vi "Add FPGA Channels.vi"(7 "error in (no error)":errorcluster, 9 "User defined IOVs":T1(array[cluster]), 10 "Item Ref in":T2 format="%.0x") -> (0 "error out":errorcluster, 3 "Item Ref out":T2 format="%.0x")   [LabVIEW 2019, in "SEECD System Explorer.lvlib"]
uses:
  SEECD System Explorer.lvlib
  <vilib>/NI VeriStand/Custom Device API/Custom Device Item Ref.ctl
  <vilib>/NI VeriStand/Custom Device API/Custom Device Channel Type.ctl
  <vilib>/NI VeriStand/Custom Device API/Custom Device API.lvlib
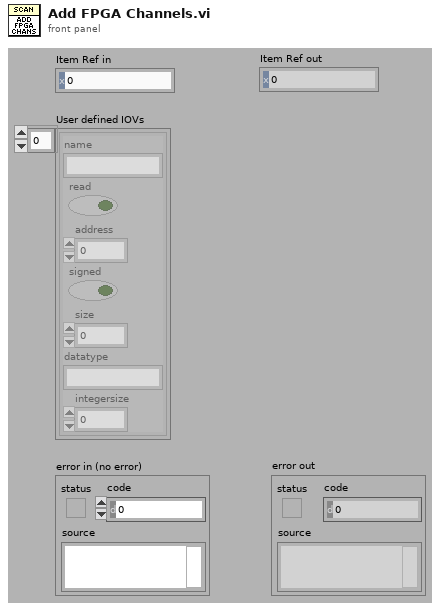
[diagram p1: front panel]
types:
  T1 = cluster{"name":string, "read":bool, "address":u32, "signed":bool, "size":u32, "datatype":string, "integersize":i32}[]
  T2 = typedef "Custom Device API.lvlib/Custom Device Item Ref.ctl" = u64
  T3 = typedef "Custom Device API.lvlib/Custom Device Channel Type.ctl" = enum16{"Input", "Output"}
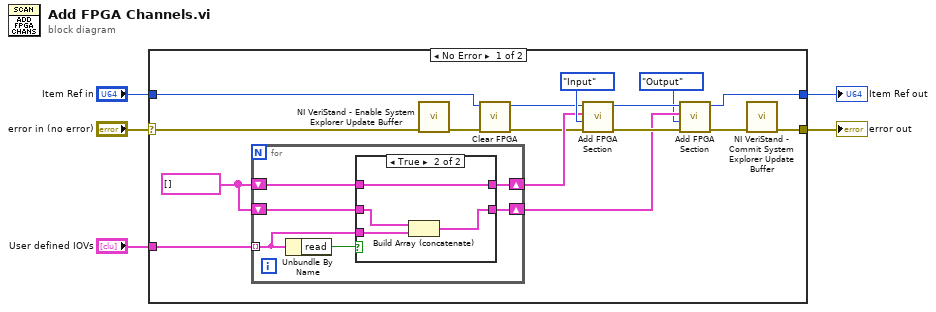
[diagram p0: block diagram]
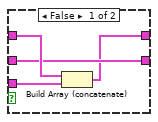
[diagram p2: hidden frame]
diagram:
  n1 = case shown="No Error" "error in (no error)" {
    selector: "error in (no error)" -> [w10 w37]
    tunnel: "User defined IOVs" -> [w21 _]
    tunnel: [w17 w36] -> w4
    tunnel: [w6 w37] -> w3
    tunnel: "Item Ref in" -> [w8 w36]
    frame No Error {
      w20 = T1 [] ("User defined IOVs")
      n2 = for {
        tunnel: w21 -> [w26] mode=indexing
        shift-right: [w22] -> w15
        shift-left: w20 -> [w24]
        shift-right: [w23] -> w14
        shift-left: w20 -> [w25]
        n3 = Unbundle By Name(w26) -> ("read"=w27:bool)
        n4 = case shown="True" w27 {
          tunnel: w26 -> [w30 w35]
          tunnel: w25 -> [w29 w34]
          tunnel: w24 -> [w31 w32]
          tunnel: [w29 w33] -> w23
          tunnel: [w28 w32] -> w22
          frame False {
            n5 = Build Array (concatenate)(w31, w30) -> (w28:T1)
          }
          frame True {
            n6 = Build Array (concatenate)(w34, w35) -> (w33:T1)
          }
        }
      }
      n7 = call <vilib>:"NI VeriStand - Enable System Explorer Update Buffer.vi"("error in (no error)"=w10) -> ("error out"=w9:errorcluster)  [unwired: 10 in]
      n8 = call "Clear FPGA.vi"("error in (no error)"=w9, "Item Ref in"=w8) -> ("error out"=w12:errorcluster, "Item Ref out"=w11:T2)  [unwired: 8 in]
      n9 = call "Add FPGA Section.vi"("error in (no error)"=w12, "Channel Type"=Custom_Device_Channel_Type."Input" ("Type"), "User defined IOVs"=w15, "Item Ref in"=w11) -> ("error out"=w19:errorcluster, "Item Ref out"=w18:T2)  [unwired: 6 in]
      n10 = call "Add FPGA Section.vi"("error in (no error)"=w19, "Channel Type"=Custom_Device_Channel_Type."Output" ("Type"), "User defined IOVs"=w14, "Item Ref in"=w18) -> ("error out"=w7:errorcluster, "Item Ref out"=w17:T2)  [unwired: 6 in]
      n11 = call <vilib>:"NI VeriStand - Commit System Explorer Update Buffer.vi"("error in (no error)"=w7) -> ("error out"=w6:errorcluster)  [unwired: 10 in]
    }
    frame Error {
    }
  }
  "Item Ref out" <- w4
  "error out" <- w3
